vi "BRig_dataBlock_c_nTrial_biasing.vi"() -> (2 "output_c_nTrial_biasing":i32)   [LabVIEW 2014]
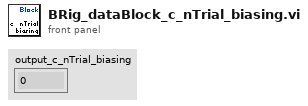
[diagram p1: front panel]
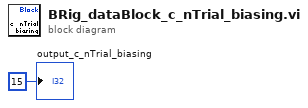
[diagram p0: block diagram]
diagram:
  "output_c_nTrial_biasing" <- 15 ("output_iBlock")
